vi "Read Temperature.vi"(8 "error in (no error)":errorcluster, 11 "TCP Network Connection in":refnum<k5>) -> (0 "error out":errorcluster, 2 "Numeric":dbl, 3 "TCP Network Connection out":refnum<k5>)   [LabVIEW 2016, in "instrument.Cryostation.lvclass"]
uses:
  instrument.Cryostation.lvclass
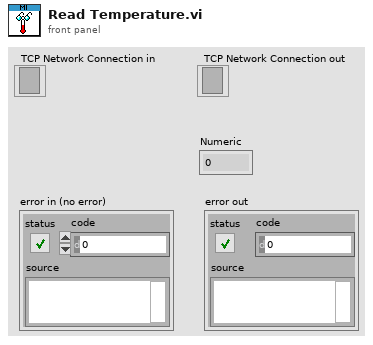
[diagram p1: front panel]
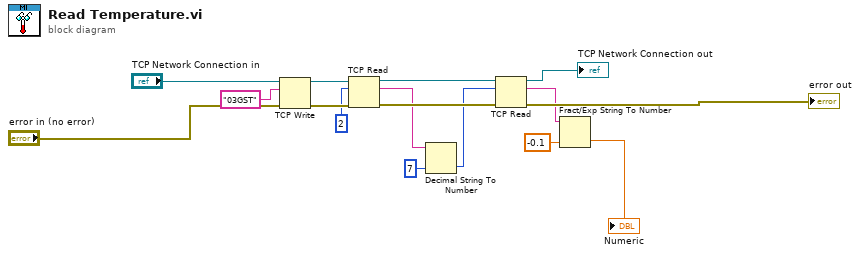
[diagram p0: block diagram]
diagram:
  n1 = TCP Write(connection ID="TCP Network Connection in", data in="03GST", error in (no error)="error in (no error)") -> (connection ID out=w4:refnum<k5>, error out=w5:errorcluster)  [unwired: 1 in, 1 out]
  n2 = TCP Read(connection ID=w4, bytes to read=2, error in (no error)=w5) -> (connection ID out=w9:refnum<k5>, data out=w6:string, error out=w10:errorcluster)  [unwired: 2 in]
  n3 = Decimal String To Number(string=w6, default (0L)=7 ("default (0 I32)")) -> (number=w8:i32)  [unwired: 1 in, 1 out]
  n4 = TCP Read(connection ID=w9, bytes to read=w8, error in (no error)=w10) -> (connection ID out=→"TCP Network Connection out":refnum<k5>, data out=w11:string, error out=→"error out":errorcluster)  [unwired: 2 in]
  n5 = Fract/Exp String To Number(string=w11, default (0 dbl)=-0.1 ("default (0 DBL)")) -> (number=→"Numeric":dbl)  [unwired: 2 in, 1 out]
